vi "Gate Until Frame Complete.vi"(0 "image metadata in":T3, 1 "reset":bool, 5 "serial channel resources":T1, 7 "serial channel selector":fxp<+,3,3>, 9 "input valid":bool, 12 "ready for output":bool) -> (4 "image metadata out":T3, 10 "output valid":bool, 14 "ready for input":bool)   [LabVIEW 2020, in "GettingStarted_Common_148X_FPGA.lvlib"]
uses:
  GettingStarted_Common_148X_FPGA.lvlib
  Types/Image Metadata.ctl
  <instrlib>/FlexRIO/CSI-2/v2/Common/Types/LLP Data Type.ctl
  Types/Serial Channel Resources.ctl
  Types/Single Serial Channel Resources.ctl
  <vilib>/rvi/DataTransferAndStorage/Container/Common/niFpgaContainerGetUniqueNameForEmu.vi
  <vilib>/rvi/DataTransferAndStorage/Container/Common/niFpgaContainerSetEmuInfo.vi
  <vilib>/rvi/eio/common/nirviEmuReportErrorAndStop.vi
  <vilib>/rvi/DataTransferAndStorage/Container/Common/niFpgaContainerExecOnDevCompGetState.vi
  <vilib>/rvi/Emulation/niFpgaEmulationIsFPGAContextNoSignature.vi
  <vilib>/rvi/Emulation/niFpgaSctlEmulationGetInTimedLoop.vi
  <vilib>/rvi/errors/niFpgaSetErrorForExecOnDevCompSimple.vi
  <vilib>/rvi/FIFO/Fifo_Resource/nirvififoEmulationSetSize.vi
  <vilib>/rvi/FIFO/Fifo_Resource/nirviFifoEmulationQueueMgr.vi
  <instcachedir>/0/nirviFifoEmulationQueueMgr_E5CAEC123FF24DC58D834DCA3CDAA9B5.lvgen/nirviFifoEmulationQueueMgr_E5CAEC123FF24DC58D834DCA3CDAA9B5_037.vi
  <vilib>/rvi/FIFO/Fifo_Resource/nirvififoEmulationDetermineInputValidOut.vi
  <vilib>/rvi/FIFO/Fifo_Resource/nirvififoEmulationCreateLock.vi
  <vilib>/rvi/Emulation/niFpgaProcessEmulError.vi
  <vilib>/rvi/FIFO/Fifo_Resource/nirvififoEmulationObtainLock.vi
  <vilib>/rvi/FIFO/Fifo_Resource/nirvififoEmulationReleaseLock.vi
  <vilib>/rvi/occurrence/nirviWaitOnOccurrenceBase.vi
  <vilib>/rvi/errors/nirviReportUnexpectedCaseInternalError.vi
  <vilib>/rvi/errors/nirviReportUnexpectedCaseInternalError (U32).vi
  <vilib>/Utility/error.llb/Clear Errors.vi
  <vilib>/rvi/interface/RandomDataEmulation/niFpgaRandomDataHandleErrors.vi
  <vilib>/rvi/LocalResourceManager/LocalResourceManager.xnode
  <vilib>/rvi/DataTransferAndStorage/Container/XNode/niFpgaContainer.xnode
  <vilib>/rvi/FIFO/Fifo_Resource/niFpgaFifoEmulationRefIn.vi
  <instrlib>/FlexRIO/CSI-2/v2/Common/NI CSI-2 API Common v2.lvlib
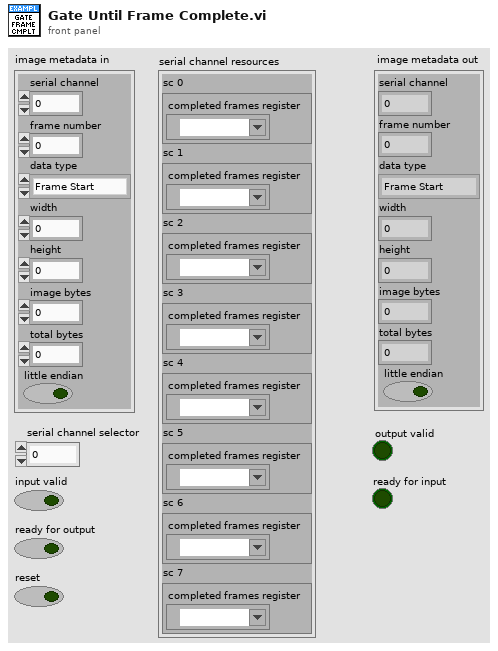
[diagram p1: front panel]
types:
  T1 = typedef "GettingStarted_Common_148X_FPGA.lvlib/Serial Channel Resources.ctl" = cluster{"sc 0":T2, "sc 1":T2, "sc 2":T2, "sc 3":T2, "sc 4":T2, "sc 5":T2, "sc 6":T2, "sc 7":T2}
  T2 = typedef "GettingStarted_Common_148X_FPGA.lvlib/Single Serial Channel Resources.ctl" = cluster{"completed frames register":refnum<k21>}
  T3 = typedef "GettingStarted_Common_148X_FPGA.lvlib/Image Metadata.ctl" = cluster{"serial channel":fxp<+,3,3>, "frame number":u16, "data type":T4, "width":u16, "height":u16, "image bytes":u32, "total bytes":u32, "little endian":bool}
  T4 = typedef "NI CSI-2 API Common v2.lvlib/LLP Data Type.ctl" = enum8{"Frame Start", "Frame End", "Line Start", "Line End", "End of Transmission", "Reserved 0", "Reserved 1", "Reserved 2", "Generic Short Packet 1", "Generic Short Packet 2", "Generic Short Packet 3", "Generic Short Packet 4", "Generic Short Packet 5", "Generic Short Packet 6", "Generic Short Packet 7", "Generic Short Packet 8", "Null", "Blanking Data", "Embedded 8-bit non Image Data", "Generic Long Packet 1", "Generic Long Packet 2", "Generic Long Packet 3", "Generic Long Packet 4", "Reserved 3", "YUV420 8-bit", "YUV420 10-bit", "Legacy YUV420 8-bit", "Reserved 4", "YUV420 8-bit Chroma Shifted", "YUV420 10-bit Chroma Shifted", "YUV422 8-bit", "YUV422 10-bit", "RGB444", "RGB555", "RGB565", "RGB666", "RGB888", "Reserved 5", "Reserved 6", "RAW 24", "RAW 6", "RAW 7", "RAW 8", "RAW 10", "RAW 12", "RAW 14", "RAW 16", "RAW 20", "User Defined 8-bit Data 1", "User Defined 8-bit Data 2", "User Defined 8-bit Data 3", "User Defined 8-bit Data 4", "User Defined 8-bit Data 5", "User Defined 8-bit Data 6", "User Defined 8-bit Data 7", "User Defined 8-bit Data 8", "USL Command", "Reserved 7", "Reserved 8", "Reserved 9", "Reserved 10", "Reserved 11", "Reserved 12", "LRTE EPD Spacer"}
  T5 = cluster{"serial channel":fxp<+,3,3>, "frame number":u16, "data type":enum8{"Frame Start", "Frame End", "Line Start", "Line End", "End of Transmission", "Reserved 0", "Reserved 1", "Reserved 2", "Generic Short Packet 1", "Generic Short Packet 2", "Generic Short Packet 3", "Generic Short Packet 4", "Generic Short Packet 5", "Generic Short Packet 6", "Generic Short Packet 7", "Generic Short Packet 8", "Null", "Blanking Data", "Embedded 8-bit non Image Data", "Generic Long Packet 1", "Generic Long Packet 2", "Generic Long Packet 3", "Generic Long Packet 4", "Reserved 3", "YUV420 8-bit", "YUV420 10-bit", "Legacy YUV420 8-bit", "Reserved 4", "YUV420 8-bit Chroma Shifted", "YUV420 10-bit Chroma Shifted", "YUV422 8-bit", "YUV422 10-bit", "RGB444", "RGB555", "RGB565", "RGB666", "RGB888", "Reserved 5", "Reserved 6", "RAW 24", "RAW 6", "RAW 7", "RAW 8", "RAW 10", "RAW 12", "RAW 14", "RAW 16", "RAW 20", "User Defined 8-bit Data 1", "User Defined 8-bit Data 2", "User Defined 8-bit Data 3", "User Defined 8-bit Data 4", "User Defined 8-bit Data 5", "User Defined 8-bit Data 6", "User Defined 8-bit Data 7", "User Defined 8-bit Data 8", "USL Command", "Reserved 7", "Reserved 8", "Reserved 9", "Reserved 10", "Reserved 11", "Reserved 12", "LRTE EPD Spacer"}, "width":u16, "height":u16, "image bytes":u32, "total bytes":u32, "little endian":bool}
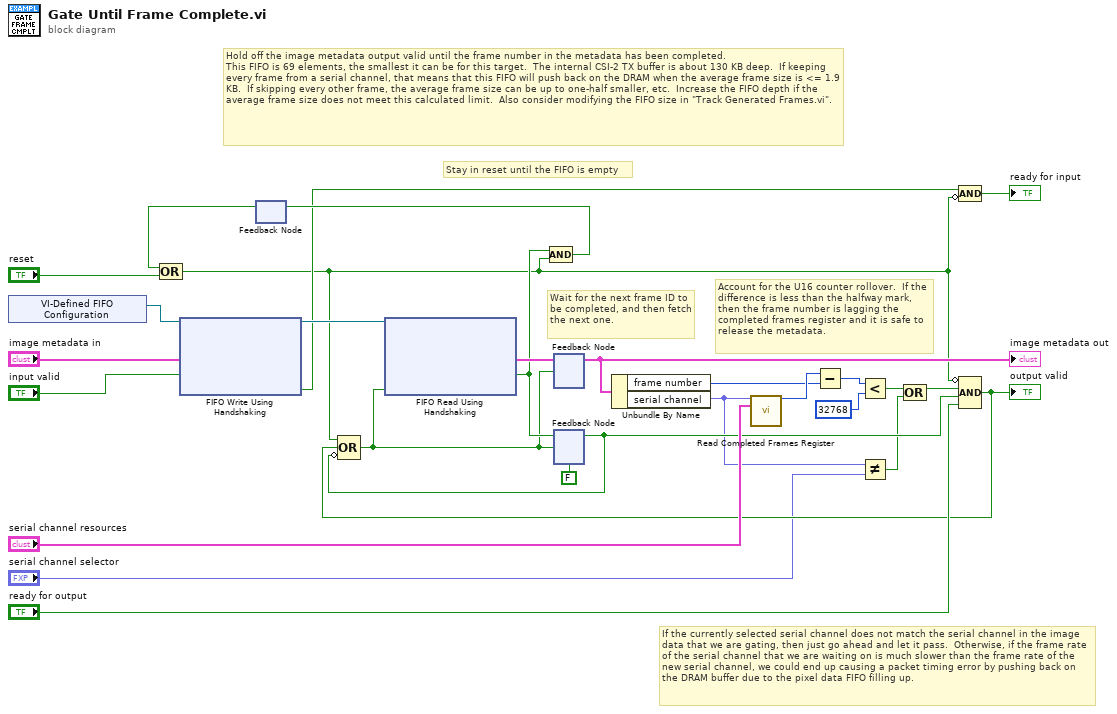
[diagram p0: block diagram]
diagram:
  # "Account for the U16 counter rollover.  If the difference is less than the halfway mark, then the frame number is lagging the completed frames register and it is safe to release the metadata."
  # "If the currently selected serial channel does not match the serial channel in the image data that we are gating, then just go ahead and let it pass.  Otherwise, if the frame rate of the serial channel that we are waiting on is much slower than the frame rate of the new serial channel, we could end up causing a packet timing error by pushing back on the DRAM buffer due to the pixel data FIFO filling up."
  # "Hold off the image metadata output valid until the frame number in the metadata has been completed.\nThis FIFO is 69 elements, the smallest it can be for this target.  The internal CSI-2 TX buffer is about 130 KB deep.  If keeping every frame from a serial channel, that means that this FIFO will push back on the DRAM when the average frame size is <= 1.9 KB.  If skipping every other frame, the average frame size can be up to one-half smaller, etc.  Increase the FIFO depth if the average frame size does not meet this calculated limit.  Also consider modifying the FIFO size in \"Track Generated Frames.vi\"."
  # "Stay in reset until the FIFO is empty"
  # "Wait for the next frame ID to be completed, and then fetch the next one."
  n1 = xnode "VI-Defined FIFO Configuration"() -> ("FIFO Out"=w27:refnum<k21>)
  n2 = xnode ("FIFO Write Using Handshaking")("Element"="image metadata in", "Input Valid"="input valid", "FIFO In"=w27) -> ("Ready for Input"=w16:bool, "FIFO Out"=w28:refnum<k21>)
  n3 = feedback #1() -> (w19:bool)  [unwired: 1 in]
  n4 = Compound Arithmetic op=OR(w19, "reset") -> (w13:bool)
  n5 = feedback #2() -> (w17:T5)  [unwired: 1 in]
  "image metadata out" <- w17
  n6 = feedback #3(FALSE ("Output Valid")) -> (w10:bool)
  n7 = Unbundle By Name(w17) -> ("frame number"=w3:u16, "serial channel"=w7:fxp<+,3,3>)
  n8 = call "Read Completed Frames Register.vi"("serial channel"=w7, "serial channel resources"="serial channel resources") -> ("completed frames"=w4:u16)  [unwired: 13 in]
  n9 = Subtract(x=w4, y=w3) -> (x-y=w2:u16)
  n10 = Less?(x=w2, y=u16 32768) -> (x < y?=w24:bool)
  n11 = Not Equal?(x=w7, y="serial channel selector") -> (x != y?=w6:bool)
  n12 = Compound Arithmetic op=OR(w24, w6) -> (w8:bool)
  n13 = Compound Arithmetic op=AND(w16, invert w13) -> (→"ready for input":bool)
  n14 = Compound Arithmetic op=AND(invert w13, w8, w10, "ready for output") -> (w9:bool)
  "output valid" <- w9
  n15 = Compound Arithmetic op=OR(w13, w9, invert w10) -> (w21:bool)
  n16 = xnode ("FIFO Read Using Handshaking")("Ready for Output"=w21, "FIFO In"=w28) -> ("Element"=w23:T5, "Output Valid"=w22:bool)  [unwired: 1 out]
  n17 = Compound Arithmetic op=AND(w22, w13) -> (w18:bool)
  n18 = feedback-in #1(w18) -> ()
  n19 = feedback-in #2(w23, w21) -> ()
  n20 = feedback-in #3(w22, w21) -> ()
